vi "Read EventLoggerDVR.vi"(8 "error in (no error)":errorcluster, 11 "EventLogger in":refnum<class "EventLogger.lvclass">) -> (0 "error out":errorcluster, 2 "EventLoggerDVR":T1, 3 "EventLogger out":refnum<class "EventLogger.lvclass">)   [LabVIEW 2015, in "EventLogger.lvclass"]
uses:
  EventLogger.lvclass
  Controls/EventLoggerDVR--DVR.ctl
  EventLogger.lvclass/EventLogger.ctl
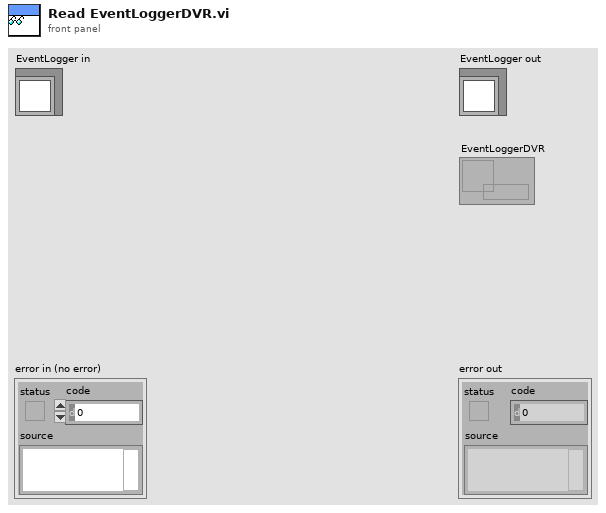
[diagram p1: front panel]
types:
  T1 = typedef "EventLoggerDVR--DVR.ctl" = refnum<data-value>
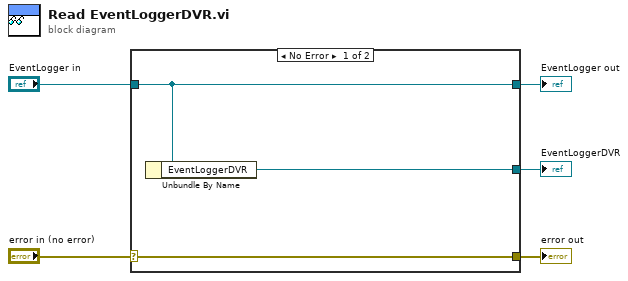
[diagram p0: block diagram]
diagram:
  n1 = case shown="No Error" "error in (no error)" {
    selector: "error in (no error)" -> [w8 w9]
    tunnel: [w8 w9] -> w4
    tunnel: [w7 w10] -> w2
    tunnel: "EventLogger in" -> [w7 w10]
    tunnel: [w6 _] -> w1
    frame No Error {
      n2 = Unbundle By Name(w7) -> ("EventLoggerDVR"=w6:T1)
    }
    frame Error {
    }
  }
  "error out" <- w4
  "EventLogger out" <- w2
  "EventLoggerDVR" <- w1
